vi "对比.vi"(8 "密码":string, 9 "密码文件":path, 10 "账户":string, 11 "账户文件":path) -> (2 "x与y？":bool)   [LabVIEW 2018]
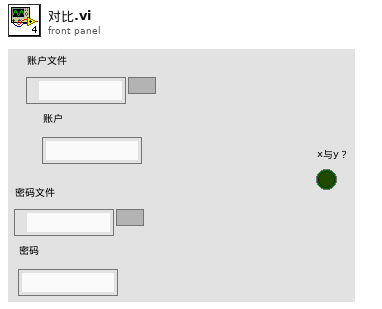
[diagram p1: front panel]
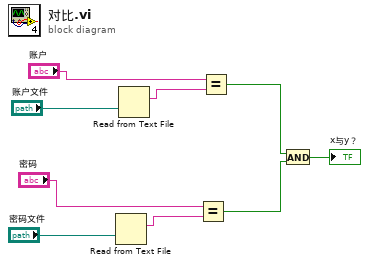
[diagram p0: block diagram]
diagram:
  n1 = Read from Text File(file (use dialog)="密码文件") -> (text=w4:string)  [unwired: 3 in, 3 out]
  n2 = Read from Text File(file (use dialog)="账户文件") -> (text=w6:string)  [unwired: 3 in, 3 out]
  n3 = Equal?(x="密码", y=w4) -> (x = y?=w2:bool)
  n4 = Equal?(x="账户", y=w6) -> (x = y?=w3:bool)
  n5 = And(x=w3, y=w2) -> (x .and. y?=→"x与y？":bool)
